vi "Eurotherm - Setup.vi"(0 "Setup In":T8 {"Min Set Point" format="%.3f"; "Max Set Point" format="%.3f"; "Communication"."Baud Rate" items=["300"=300, "600"=600, "1200"=1200, "2400"=2400, "4800"=4800, "9600 (default)"=9600, "19200"=19200, "38400"=38400, "57600"=57600, "76800"=76800, "115200"=115200, "230400"=230400]; "Communication"."Com Port" min=1 max=255; "Communication"."Address" min=1 max=99}, 7 "Action":enum16{"Read", "Write"}(ring), 9 "Index":i32=-1, 11 "error in (no error)":errorcluster) -> (4 "Setup Out":T8 {"Min Set Point" format="%.3f"; "Max Set Point" format="%.3f"; "Communication"."Baud Rate" items=["300"=300, "600"=600, "1200"=1200, "2400"=2400, "4800"=4800, "9600 (default)"=9600, "19200"=19200, "38400"=38400, "57600"=57600, "76800"=76800, "115200"=115200, "230400"=230400]; "Communication"."Com Port" min=1 max=255; "Communication"."Address" min=1 max=99}, 6 "Setup Out":T1={"Communication"={"Com Port"=1, "Address"=1, "Baud Rate"=9600}, "Name"="", "Enable"=FALSE, "Max Set Point"=0.0, "Min Set Point"=0.0, "Units"="", "Graph Data"=0, "Sensor type"=enum."RhFe", "Calibration File Path"=path "", "Conversion Type"=enum."Linear"} {"Min Set Point" format="%.3f"; "Max Set Point" format="%.3f"; "Communication"."Baud Rate" items=["300"=300, "600"=600, "1200"=1200, "2400"=2400, "4800"=4800, "9600 (default)"=9600, "19200"=19200, "38400"=38400, "57600"=57600, "76800"=76800, "115200"=115200, "230400"=230400]; "Communication"."Com Port" min=1 max=255; "Communication"."Address" min=1 max=99}, 15 "error out":errorcluster)   [LabVIEW 2011]
uses:
  Eurotherm - Controls/Eurotherm - Setups.ctl
  Eurotherm - Controls/Eurotherm - Setup.ctl
  Eurotherm - Controls/Eurotherm - Communication.ctl
  Common/Utilities/Controls - Com Ports/Com Port - Numeric.ctl
  Eurotherm - Controls/Eurotherm - Address.ctl
  Common/Utilities/Controls - Com Ports/Com Port - Baud Rate.ctl
  Common/Utilities - System/Sensors/Sensors - Controls/Sensors - Temperature Sensor Type.ctl
  Common/Utilities - System/Sensors/Sensors - Controls/Sensors - Conversion Type.ctl
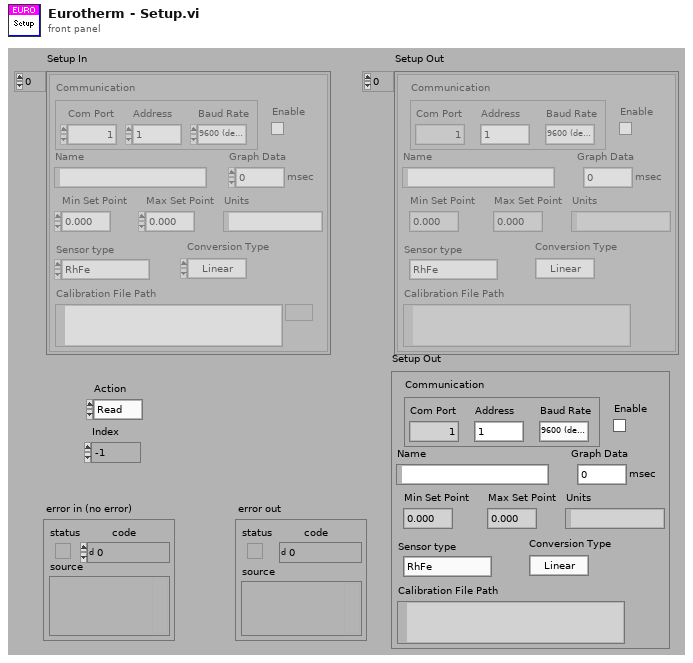
[diagram p1: front panel]
types:
  T1 = typedef "Eurotherm - Setup.ctl" = cluster{"Communication":T2, "Name":string, "Enable":bool, "Max Set Point":dbl, "Min Set Point":dbl, "Units":string, "Graph Data":u32, "Sensor type":T6, "Calibration File Path":path, "Conversion Type":T7}
  T2 = typedef "Eurotherm - Communication.ctl" = cluster{"Com Port":T3, "Address":T4, "Baud Rate":T5}
  T3 = typedef "Com Port - Numeric.ctl" = i32
  T4 = typedef "Eurotherm - Address.ctl" = u8
  T5 = typedef "Com Port - Baud Rate.ctl" = u32
  T6 = typedef "Sensors - Temperature Sensor Type.ctl" = enum16{"RhFe", "Pt", "K type thermocouple", "W5 type thermocouple", "No Conversion"}
  T7 = typedef "Sensors - Conversion Type.ctl" = enum16{"Linear", "Spline"}
  T8 = typedef "Eurotherm - Setups.ctl" = T1[]
  T9 = enum16{"read/write", "read-only", "write-only", "write-only (truncate)"}
  T10 = enum16{"open", "replace", "create", "open or create", "replace or create", "replace or create with confirmation"}
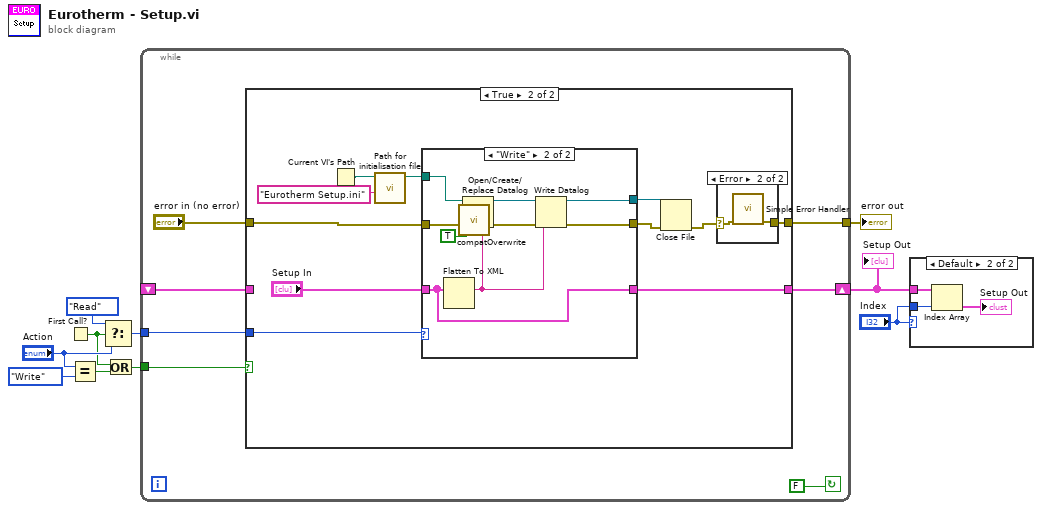
[diagram p0: block diagram]
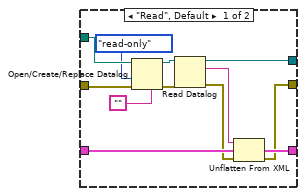
[diagram p4: hidden frame]
diagram:
  n1 = First Call?() -> (First Call?: T/F=w5:bool)
  n2 = Equal?(x="Action", y=enum16{"Read", "Write"}."Write") -> (x = y?=w4:bool)
  n3 = Select(t=enum16{"Read", "Write"}."Read" ("Action"), s=w5, f="Action") -> (s? t:f=w9:enum16{"Read", "Write"})
  n4 = Or(x=w5, y=w4) -> (x .or. y?=w6:bool)
  n5 = while {
    tunnel: w9 -> [w17]
    shift-right: [w16] -> w1
    shift-left: _ -> [w14]
    tunnel: w6 -> [w13]
    tunnel: [w12] -> w3
    stop <- FALSE continue-if-true
    n6 = case shown="True" w13 {
      tunnel: w17 -> [_ w26]
      tunnel: [w19 w28] -> w16
      tunnel: w14 -> [w19 _]
      tunnel: [w18 w30] -> w12
      tunnel: "error in (no error)" -> [w18 w29]
      frame False {
      }
      frame True {
        n7 = Current VI's Path() -> (path=w22:path)
        n8 = call "Path for initialisation file.vi"("Init File Name"="Eurotherm Setup.ini", "VI Path"=w22) -> ("Required Path"=w20:path)  [unwired: 9 in]
        n9 = case shown="\"Write\"" w26 {
          tunnel: [w42 w48] -> w24
          tunnel: [w32 w52] -> w25
          tunnel: [w34 w44] -> w28
          tunnel: w20 -> [w41 w51]
          tunnel: "Setup In" -> [w35 w44]
          tunnel: w29 -> [w38 w46]
          frame "Read", Default {
            n10 = Open/Create/Replace Datalog(5:"", 8:w38, 9:T9."read-only" ("open mode (0)"), 11:w41) -> (0:w39:errorcluster, 3:w40:refnum<k1>)  [unwired: 2 in, 1 out]
            n11 = Read Datalog(4:w39, 7:w40) -> (0:w33:errorcluster, 2:w31:string, 3:w42:refnum<k1>)  [unwired: 1 in]
            n12 = Unflatten From XML(xml string=w31, type=w35, error in (no error)=w33) -> (value=w34:T8, error out=w32:errorcluster)
          }
          frame "Write" {
            n13 = Flatten To XML(anything=w44) -> (xml string=w45:string)
            n14 = call <vilib>:"compatOverwrite.vi"("overwrite (F)"=TRUE) -> ("overwrite?"=w43:T10)
            n15 = Open/Create/Replace Datalog(5:w45, 8:w46, 10:w43, 11:w51) -> (0:w49:errorcluster, 3:w50:refnum<k1>)  [unwired: 2 in, 1 out]
            n16 = Write Datalog(4:w49, 6:w45, 7:w50) -> (0:w52:errorcluster, 3:w48:refnum<k1>)
          }
        }
        n17 = Close File(refnum=w24, error in=w25) -> (error out=w23:errorcluster)  [unwired: 1 out]
        n18 = case shown="Error" w23 {
          selector: w23 -> [w53 w54]
          tunnel: [w53 w55] -> w30
          frame No Error {
          }
          frame Error {
            n19 = call <vilib>:"Simple Error Handler.vi"("error in (no error)"=w54) -> ("error out"=w55:errorcluster)  [unwired: 4 in, 4 out]
          }
        }
      }
    }
  }
  "error out" <- w3
  "Setup Out" <- w1
  n20 = case shown="Default" "Index" {
    tunnel: w1 -> [_ w58]
    tunnel: "Index" -> [_ w57]
    frame -1 {
    }
    frame Default {
      n21 = Index Array(array=w58, index=w57) -> (element=→"Setup Out":T1)
    }
  }
